vi "Create Instrument SMO.vi"(8 "error in (no error)":errorcluster, 9 "Debug Mode? [F]":bool, 10 "Configuration Window? [T]":bool=TRUE, 11 "Instrument in":refnum<class "Instrument.lvclass">) -> (0 "error out":errorcluster, 3 "Instrument out":refnum<class "Instrument.lvclass">)   [LabVIEW 2019, in "Instrument.lvclass"]
doc: "Create a new instance of your Instrument. A little bt of configuration happens before calling \"Create SMO.vi\""
uses:
  Instrument.lvclass
  C:/Program Files (x86)/National Instruments/LabVIEW 2019/vi.lib/JKI/JKI SMO/SMO/SMO.lvclass
  Instrument.lvclass/Instrument.ctl
  <vilib>/JKI/JKI SMO/SMO/SMO.lvclass
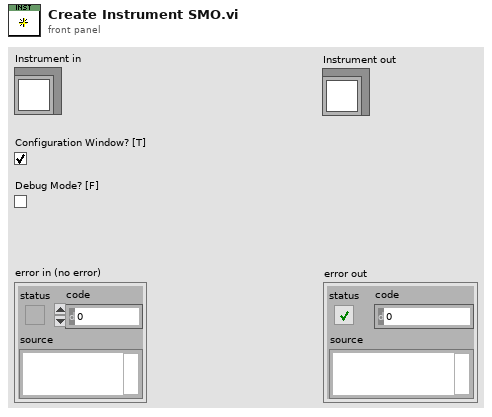
[diagram p1: front panel]
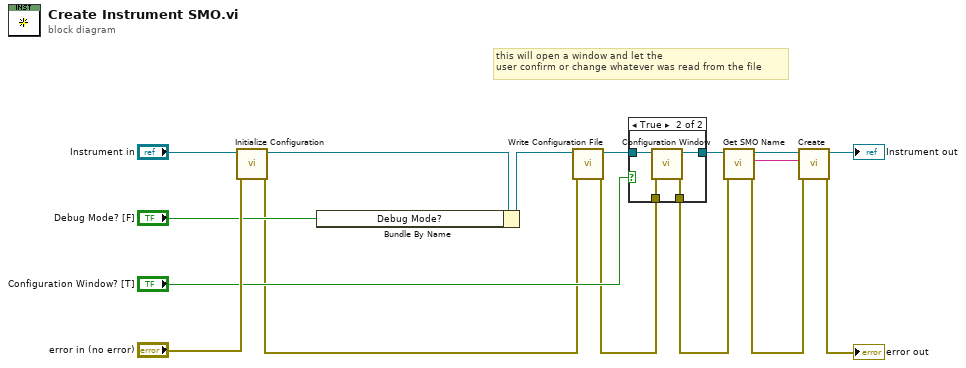
[diagram p0: block diagram]
diagram:
  # "this will open a window and let the\nuser confirm or change whatever was read from the file"
  n1 = call "Initialize Configuration.vi"("error in (no error)"="error in (no error)", "Instrument in"="Instrument in") -> ("error out"=w3:errorcluster, "Instrument out"=w6:refnum<class "Instrument.lvclass">)  [unwired: 8 in]
  n2 = Bundle By Name(cluster=w6, "Debug Mode?"="Debug Mode? [F]") -> (w4:refnum<class "Instrument.lvclass">)
  n3 = call-dynamic "Write Configuration File.vi"("error in (no error)"=w3, "Instrument in"=w4) -> ("error out"=w2:errorcluster, "Instrument out"=w1:refnum<class "Instrument.lvclass">)  [unwired: 8 in]
  n4 = case shown="True" "Configuration Window? [T]" {
    tunnel: [w17 w22] -> w10
    tunnel: [w18 w21] -> w11
    tunnel: w1 -> [w18 w20]
    tunnel: w2 -> [w17 w19]
    frame False {
    }
    frame True {
      n5 = call-dynamic "Configuration Window.vi"("error in (no error)"=w19, "Instrument"=w20) -> ("error out"=w22:errorcluster, "Instrument out"=w21:refnum<class "Instrument.lvclass">)  [unwired: 8 in]
    }
  }
  n6 = call-dynamic "Get SMO Name.vi"("error in (no error)"=w10, "Instrument in"=w11) -> ("error out"=w8:errorcluster, "SMO Name"=w7:string, "Instrument out"=w9:refnum<class "Instrument.lvclass">)  [unwired: 7 in]
  n7 = call <vilib>:"Create.vi"("error in (no error)"=w8, "Subsystem Name (optional)"=w7, "SMO"=w9) -> ("error out"=→"error out":errorcluster, "SMO out"=→"Instrument out":refnum<class "Instrument.lvclass">)  [unwired: 6 in, 1 out]
